vi "Rollback Transaction.vi"(8 "error in (no error)":errorcluster, 11 "DbConnection in":refnum<class "DbConnection.lvclass">) -> (0 "error out":errorcluster, 3 "DbConnection out":refnum<class "DbConnection.lvclass">)   [LabVIEW 2020, in "ORM.lvlib" / "DbConnection.lvclass"]
uses:
  DbConnection.lvclass
  DbConnection.lvclass/DbConnection.ctl
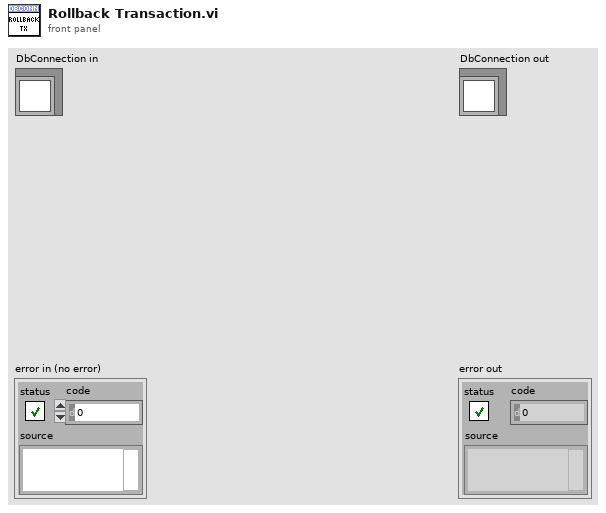
[diagram p1: front panel]
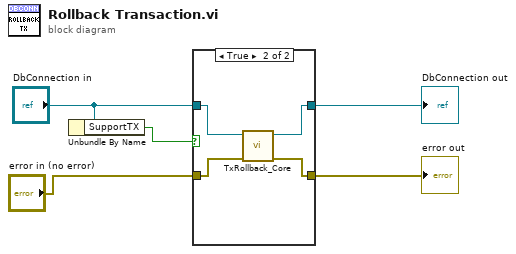
[diagram p0: block diagram]
diagram:
  n1 = Unbundle By Name("DbConnection in") -> ("SupportTX"=w2:bool)
  n2 = case shown="True" w2 {
    tunnel: [w7 w10] -> w5
    tunnel: [w6 w8] -> w4
    tunnel: "DbConnection in" -> [w7 w11]
    tunnel: "error in (no error)" -> [w6 w9]
    frame False {
    }
    frame True {
      n3 = call "TxRollback_Core.vi"("error in (no error)"=w9, "DbConnection in"=w11) -> ("error out"=w8:errorcluster, "DbConnection out"=w10:refnum<class "DbConnection.lvclass">)  [unwired: 8 in]
    }
  }
  "error out" <- w4
  "DbConnection out" <- w5
